vi "regGenToServerUserEvent.vi"(8 "error in (no error)":errorcluster, 11 "TcpServerBase in":refnum<class "TcpServerBase.lvclass">) -> (0 "error out":errorcluster, 3 "TcpServerBase out":refnum<class "TcpServerBase.lvclass">)   [LabVIEW 2018, in "TcpServerBase.lvclass"]
doc: "Register the GenToServer user event."
uses:
  TcpServerBase.lvclass
  TcpServerBase.lvclass/TcpServerBase.ctl
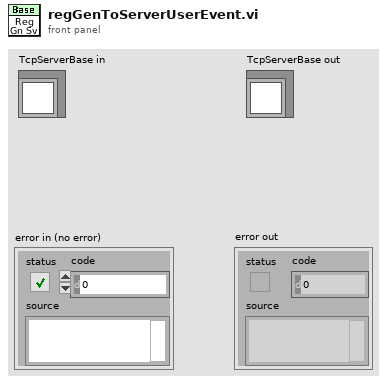
[diagram p1: front panel]
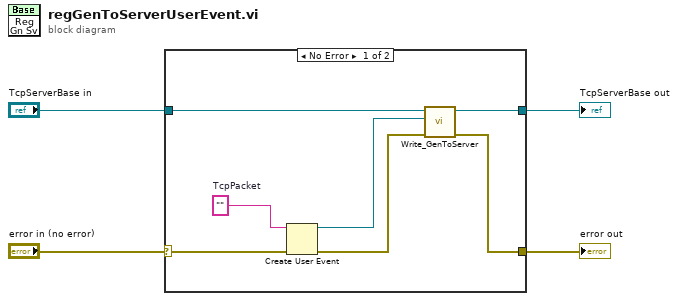
[diagram p0: block diagram]
diagram:
  n1 = case shown="No Error" "error in (no error)" {
    selector: "error in (no error)" -> [w9 w12]
    tunnel: "TcpServerBase in" -> [w11 w13]
    tunnel: [w10 w13] -> w3
    tunnel: [w7 w12] -> w1
    frame No Error {
      w6 = ""  # TcpPacket
      n2 = Create User Event(user event datatype=w6, error in=w9) -> (user event=w5:refnum<user-event>, error out=w8:errorcluster)
      n3 = call "Write_GenToServer.vi"("error in (no error)"=w8, "GenToServer"=w5, "TcpServerBase in"=w11) -> ("error out"=w7:errorcluster, "TcpServerBase out"=w10:refnum<class "TcpServerBase.lvclass">)  [unwired: 7 in]
    }
    frame Error {
    }
  }
  "TcpServerBase out" <- w3
  "error out" <- w1
